vi "Remap EOLN.vi"(0 "string in":string, 1 "line separator (\\r\\n)":string="\r\n") -> (2 "string out":string)   [LabVIEW 2014]
doc: "Replaces all EOLN characters in the string with \"line separator\"."
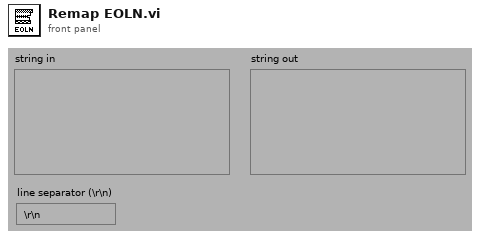
[diagram p1: front panel]
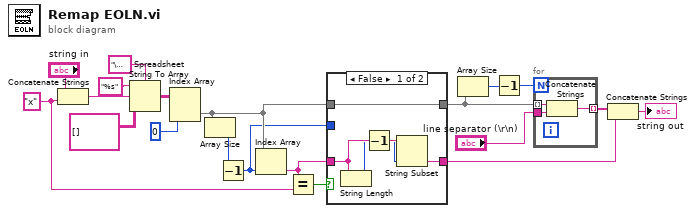
[diagram p0: block diagram]
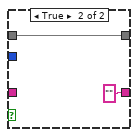
[diagram p2: hidden frame]
diagram:
  w13 = "x"
  n1 = Concatenate Strings("string in", w13) -> (w14:string)
  n2 = Spreadsheet String To Array(delimiter (Tab)="\u0000", format string="%s", spreadsheet string=w14, array type (2D Dbl)=string[][] []) -> (array=w17:string[][])
  n3 = Index Array(array=w17, index (col)=0) -> (element=w12:string[])  [unwired: 1 in]
  n4 = Array Size(array=w12) -> (size(s)=w8:i32)
  n5 = Decrement(x=w8) -> (x-1=w11:i32)
  n6 = Index Array(array=w12, index=w11) -> (element=w10:string)
  n7 = Equal?(x=w10, y=w13) -> (x = y?=w9:bool)
  n8 = case shown="False" w9 {
    tunnel: w12 -> [w22 w27]
    tunnel: [w22 w27] -> w6
    tunnel: w11 -> [_ _]
    tunnel: w10 -> [w25 _]
    tunnel: [w21 "" ("substring")] -> w3
    frame False {
      n9 = String Length(string=w25) -> (length=w24:i32)
      n10 = Decrement(x=w24) -> (x-1=w23:i32)
      n11 = String Subset(string=w25, length (rest)=w23) -> (substring=w21:string)  [unwired: 1 in]
    }
    frame True {
    }
  }
  n12 = Array Size(array=w6) -> (size(s)=w7:i32)
  n13 = Decrement(x=w7) -> (x-1=w2:i32)
  n14 = for {
    N: w2 -> [_]
    tunnel: w6 -> [w30] mode=indexing
    tunnel: "line separator (\\r\\n)" -> [w29]
    tunnel: [w28] -> w5 mode=indexing
    n15 = Concatenate Strings(w30, w29) -> (w28:string)
  }
  n16 = Concatenate Strings(w5, w3) -> (→"string out":string)
